vi "5.10 Color Threshold.vi"(0 "Input Fuzzy Blue Threshold":i32=120, 2 "Resample Scaling":i32=20, 3 "Buffers In":T2) -> (1 "Buffers Out":T2)   [LabVIEW 2011]
uses:
  5.10 Buffers Cluster.ctl
  <vilib>/userdefined/High Color/IMAQdx.ctl
  <vilib>/vision/Image Controls.llb/IMAQ Image.ctl
  <vilib>/vision/NI_Vision_Development_Module.lvlib
panel:
  out "Re-Mapping":T1(plugin-control)
  out "Plane":T1(plugin-control)
  out "Resample":T1(plugin-control)
  out "Raw":T1(plugin-control)
  out "Lookup Function":u8[](graph)
  out "User Lookup":u8[](array[numeric])=[0, 20, 40]
  in  "error out":errorcluster
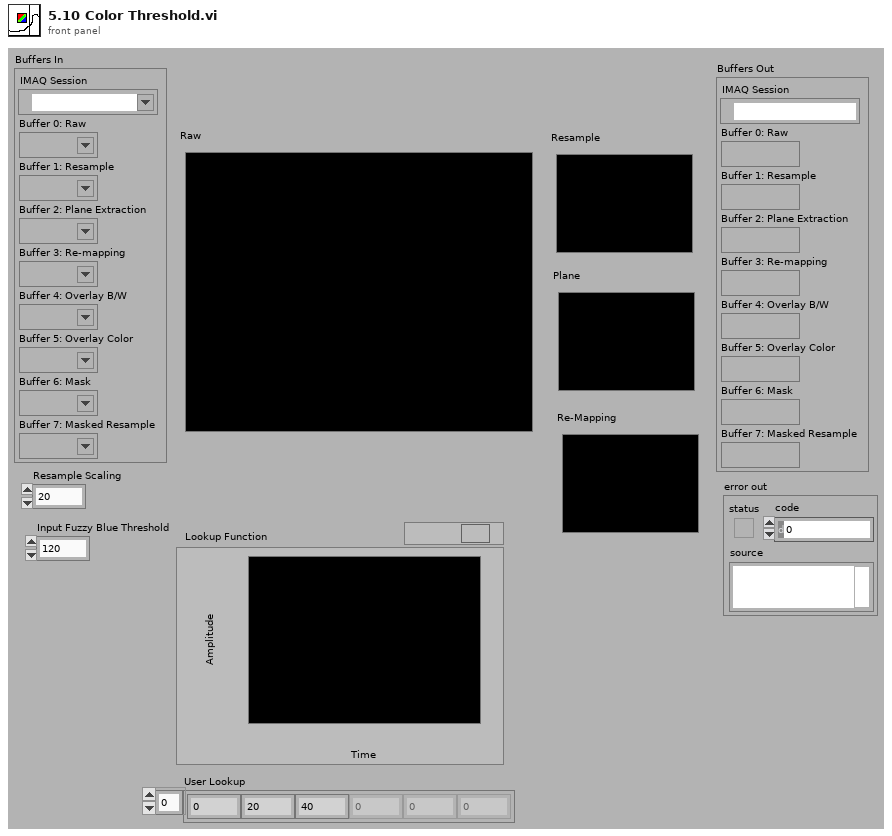
[diagram p1: front panel]
types:
  T1 = typedef "IMAQ Image.ctl" = refnum<image>
  T2 = typedef "5.10 Buffers Cluster.ctl" = cluster{"IMAQ Session":T3, "Buffer 0: Raw":T1, "Buffer 1: Resample":T1, "Buffer 2: Plane Extraction":T1, "Buffer 3: Re-mapping":T1, "Buffer 4: Overlay B/W":T1, "Buffer 5: Overlay Color":T1, "Buffer 6: Mask":T1, "Buffer 7: Masked Resample":T1}
  T3 = typedef "IMAQdx.ctl" = refnum<k21>
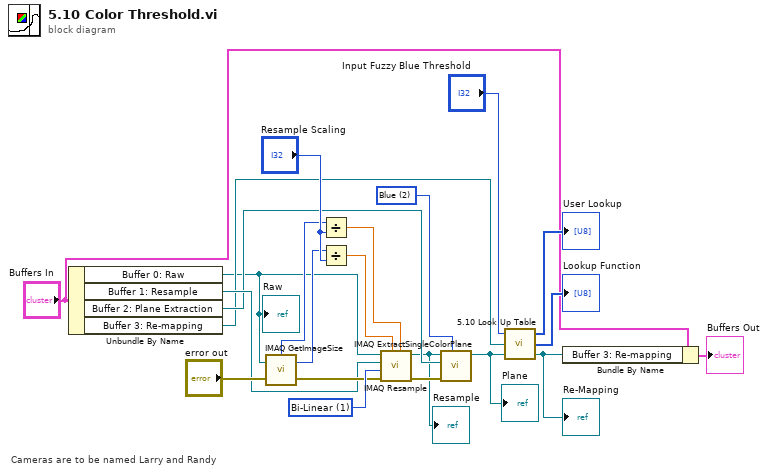
[diagram p0: block diagram]
diagram:
  w12 = 2 items=["Red", "Green", "Blue", "Hue", "Saturation", "Luminance", "Value", "Intensity"] ("Color Plane")
  w18 = u32 1 items=["Zero Order", "Bi-Linear", "Quadratic", "Cubic Spline"] ("Interpolation Type")
  # "Cameras are to be named Larry and Randy"
  n1 = Unbundle By Name("Buffers In") -> ("Buffer 0: Raw"=w3:T1, "Buffer 1: Resample"=w9:T1, "Buffer 2: Plane Extraction"=w8:T1, "Buffer 3: Re-mapping"=w7:T1)
  "Raw" <- w3
  n2 = call "IMAQ GetImageSize"("Image"=w3, "error in (no error)"="error out") -> ("Y Resolution"=w20:i32, "X Resolution"=w21:i32, "error out"=w17:errorcluster)  [unwired: 2 in]
  n3 = Divide(x=w21, y="Resample Scaling") -> (x/y=w1:dbl)
  n4 = Divide(x=w20, y="Resample Scaling") -> (x/y=w2:dbl)
  n5 = call "IMAQ Resample"("X Resolution"=w1, "Y Resolution"=w2, "error in (no error)"=w17, "Interpolation Type"=w18, "Image Dst"=w9, "Image Src"=w3) -> ("error out"=w16:errorcluster, "Image Dst Out"=w6:T1)  [unwired: 4 in]
  "Resample" <- w6
  n6 = call "IMAQ ExtractSingleColorPlane"("Color Plane"=w12, "error in (no error)"=w16, "Image Dst"=w8, "Image Src"=w6) -> ("Image Dst Out"=w5:T1)  [unwired: 6 in, 1 out]
  "Plane" <- w5
  n7 = call "5.10 Look Up Table.vi"("Image Dst Out 2"=w5, "Output Buffer"=w7, "Input Fuzzy Blue Threshold"="Input Fuzzy Blue Threshold") -> ("Image Dst Out"=w4:T1, "Lookup Table"=→"Lookup Function":u8[], "User Lookup"=→"User Lookup":u8[])
  "Re-Mapping" <- w4
  n8 = Bundle By Name(cluster="Buffers In", "Buffer 3: Re-mapping"=w4) -> (→"Buffers Out":T2)
